vi "Create Evaluation String.vi"(8 "error in (no error)":errorcluster, 10 "Evaluation String":string, 11 "Floating Point in":refnum<class "Floating Point.lvclass">) -> (0 "error out":errorcluster, 3 "Floating Point out":refnum<class "Floating Point.lvclass">)   [LabVIEW 2018, in "Floating Point.lvclass"]
uses:
  Floating Point.lvclass
  Test.lvclass
  C:/Users/UKHornP/Documents/Work/Projects/Assert_API/Plugins/Utility/Test Classes/Test.lvclass
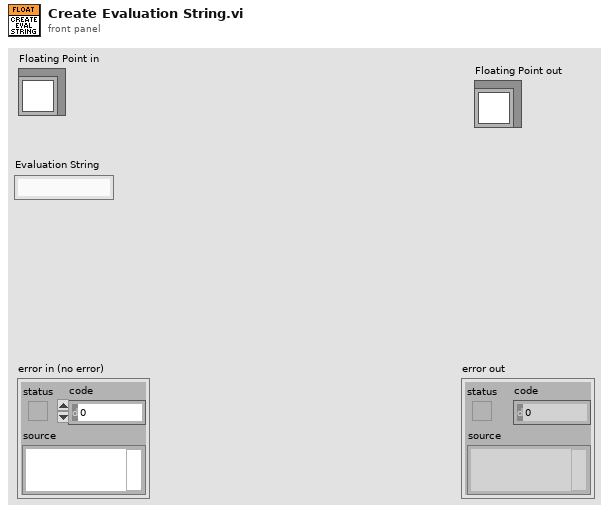
[diagram p1: front panel]
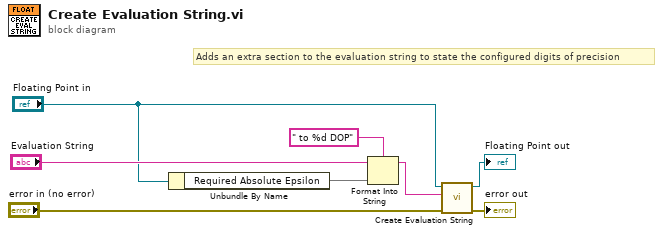
[diagram p0: block diagram]
diagram:
  # "Adds an extra section to the evaluation string to state the configured digits of precision"
  n1 = Unbundle By Name("Floating Point in") -> ("Required Absolute Epsilon"=w5)
  n2 = Format Into String(format string=" to %d DOP", initial string="Evaluation String", w5) -> (resulting string=w1:string)  [unwired: 1 in, 1 out]
  n3 = call-parent "Create Evaluation String.vi"("error in (no error)"="error in (no error)", "Evaluation String"=w1, "Test in"="Floating Point in") -> ("error out"=→"error out":errorcluster, "Test out"=→"Floating Point out":refnum<class "Floating Point.lvclass">)  [unwired: 7 in]
